vi "Sensirion SHT25 - VISA blink.vi"(8 "Error In":errorcluster, 11 "VISA in":refnum<visa-resource-name>) -> (0 "Error Out":errorcluster, 3 "VISA out":refnum<visa-resource-name>)   [LabVIEW 2012]
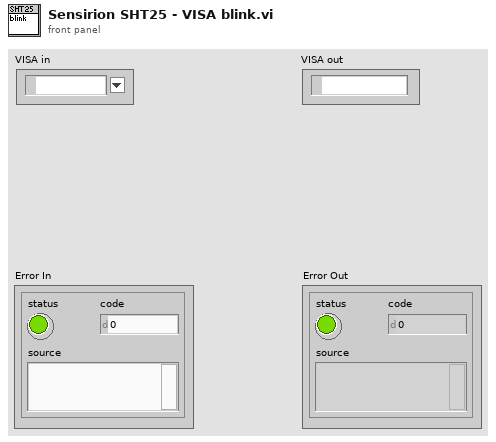
[diagram p1: front panel]
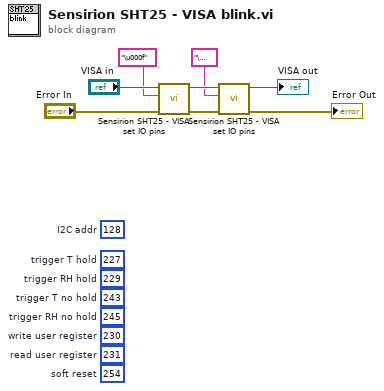
[diagram p0: block diagram]
diagram:
  (unwired) u8 254  # soft reset
  (unwired) u8 231  # read user register
  (unwired) u8 230  # write user register
  (unwired) u8 245  # trigger RH no hold
  (unwired) u8 243  # trigger T no hold
  (unwired) u8 229  # trigger RH hold
  (unwired) u8 128  # I2C addr
  (unwired) u8 227  # trigger T hold
  n1 = call "Sensirion SHT25 - VISA set IO pins.vi"("Error In"="Error In", "I/O pins"="\u000f", "VISA in"="VISA in") -> ("Error Out"=w3:errorcluster, "VISA out"=w5:refnum<visa-resource-name>)  [unwired: 6 in, 1 out]
  n2 = call "Sensirion SHT25 - VISA set IO pins.vi"("Error In"=w3, "I/O pins"="\u000e", "VISA in"=w5) -> ("Error Out"=→"Error Out":errorcluster, "VISA out"=→"VISA out":refnum<visa-resource-name>)  [unwired: 6 in, 1 out]
